vi "I2C FPGA.vi"() -> ()   [LabVIEW 2017]
uses:
  <vilib>/IEDriver/SPIandI2C/FPGA/Library/IP SPI&I2C.lvlib
  <vilib>/IEDriver/SPIandI2C/FPGA/Private/Configure Port (I2C).vi
  <vilib>/IEDriver/SPIandI2C/FPGA/Private/Read Port (I2C).vi
  <vilib>/IEDriver/SPIandI2C/FPGA/Private/Arm Port (I2C).vi
  <vilib>/IEDriver/SPIandI2C/FPGA/Private/Write Port (I2C).vi
  <vilib>/IEDriver/SPIandI2C/FPGA/Private/Initialize Port (I2C).vi
  <vilib>/IEDriver/SPIandI2C/FPGA/Private/IP Port (I2C).vi
  <vilib>/eio/EIONode/EIONode.xnode
  <vilib>/rvi/eio/common/nirviEmuTemplateMethod_errors.vi
panel:
  in  "I2C Protocol Action 0":T1(ring)=enum."Idle"
  in  "I2C Protocol Input Data 0":u8
  out "I2C Protocol Output Data 0":u8
  in  "I2C Protocol Configure 0":T2 {"Command (Write & Read)" items=["Write & Read", "Write", "Read"]}
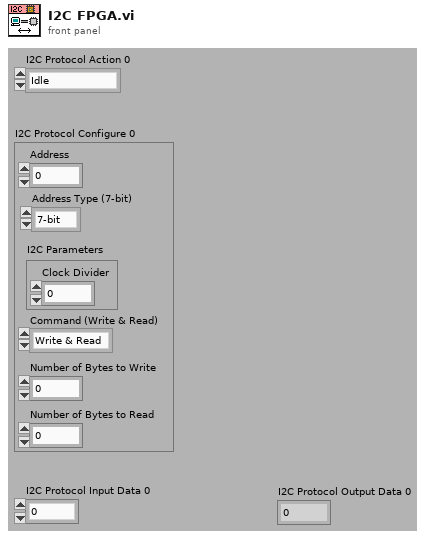
[diagram p1: front panel]
types:
  T1 = enum8{"Configure", "Write", "Arm", "Read", "Set Idle", "Idle"}
  T2 = cluster{"Address":u16, "Address Type (7-bit)":enum16{"7-bit", "10-bit"}, "I2C Parameters":cluster{"Clock Divider":u32}, "Command (Write & Read)":u8, "Number of Bytes to Write":u16, "Number of Bytes to Read":u16}
  T3 = typedef "IP SPI&I2C.lvlib/Private Data (I2C).ctl" = cluster{"Arm Trigger":refnum<k21>, "API to IP Data":refnum<k21>, "IP to API Data":refnum<k21>, "Configuration Register":refnum<k21>, "Configuration Lock":refnum<k21>}
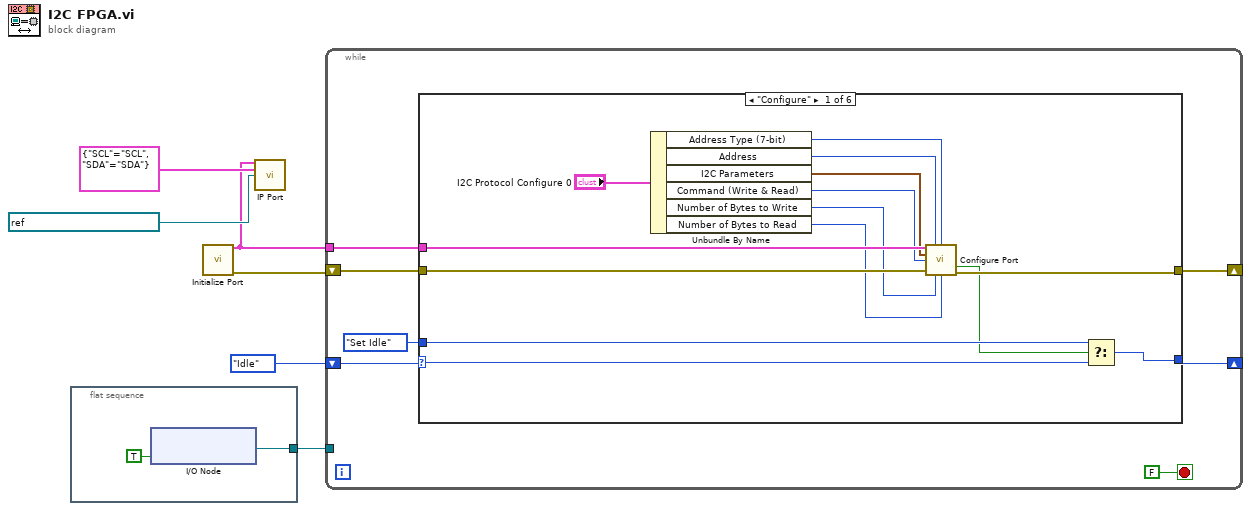
[diagram p0: block diagram]
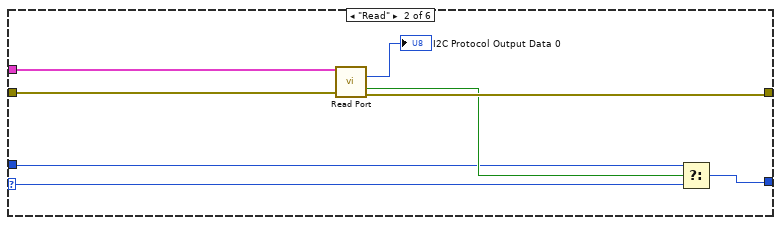
[diagram p2: hidden frame]
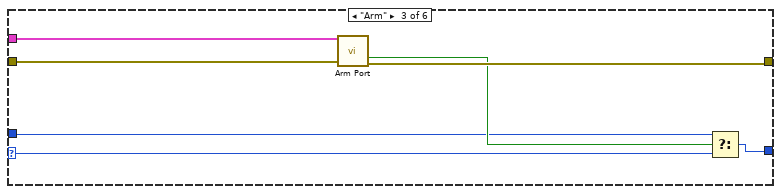
[diagram p3: hidden frame]
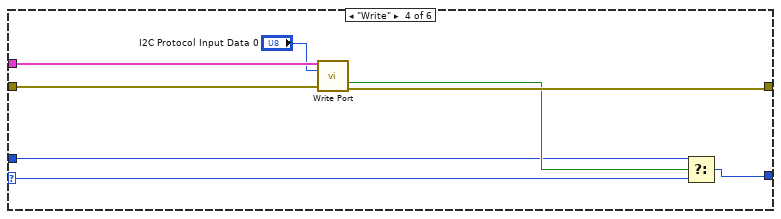
[diagram p4: hidden frame]
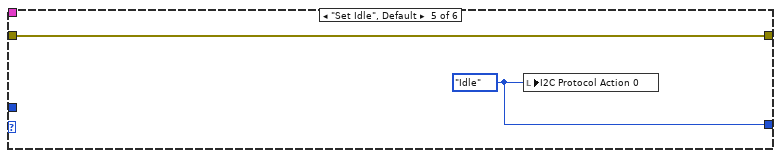
[diagram p5: hidden frame]
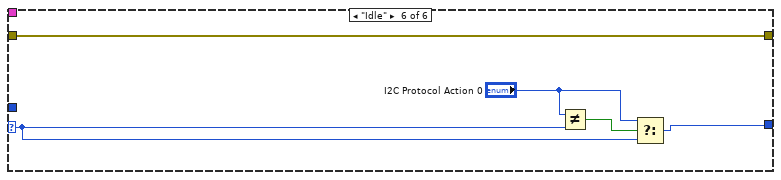
[diagram p6: hidden frame]
diagram:
  n1 = flat-sequence {
    tunnel: [w7] -> w1
    frame #0 {
      n2 = xnode "I/O Node"("Mod1/DIO1"=TRUE) -> ("FPGA I/O Out"=w7:refnum<k21>)  [unwired: 1 in]
    }
  }
  n3 = call-poly <vilib>:"Initialize Port.vi"() -> ("Private Data Out"=w4:T3, "error out"=w3:errorcluster)  [unwired: 14 in]
  n4 = call-poly <vilib>:"IP Port.vi"("Private Data In"=w4, "I2C FPGA IO"=cluster{"SCL":refnum<k21>, "SDA":refnum<k21>} {"SCL"="SCL", "SDA"="SDA"}, "FPGA Clock"=refnum<k21> "40 MHz Onboard Clock") -> ()  [unwired: 13 in]
  n5 = while {
    shift-right: [w12] -> _
    shift-left: w3 -> [w14]
    tunnel: w4 -> [w15]
    shift-right: [w10] -> _
    shift-left: T1."Idle" ("Action") -> [w11]
    tunnel: w1 -> [_]
    stop <- FALSE stop-if-true
    n6 = case shown="\"Configure\"" w11 {
      selector: w11 -> [w20 w31 w39 w46 _ w56]
      tunnel: w15 -> [w29 w37 w44 w52 _ _]
      tunnel: w14 -> [w28 w36 w43 w51 w54 w59]
      tunnel: [w27 w35 w42 w50 w54 w59] -> w12
      tunnel: [w21 w33 w41 w47 w53 w55] -> w10
      tunnel: T1."Set Idle" ("Action") -> [w19 w30 w38 w45 _ _]
      frame "Configure" {
        n7 = Unbundle By Name("I2C Protocol Configure 0") -> ("Address Type (7-bit)"=w25:enum16{"7-bit", "10-bit"}, "Address"=w16:u16, "I2C Parameters"=w24:cluster{"Clock Divider":u32}, "Command (Write & Read)"=w17:u8, "Number of Bytes to Write"=w23:u16, "Number of Bytes to Read"=w22:u16)
        n8 = call-poly <vilib>:"Configure Port.vi"("Private Data In"=w29, "Address"=w16, "Address Type (7-bit)"=w25, "I2C Parameters"=w24, "Command (Write & Read)"=w17, "error in"=w28, "Number of Bytes to Write"=w23, "Number of Bytes to Read"=w22) -> ("Done"=w18:bool, "error out"=w27:errorcluster)  [unwired: 5 in, 1 out]
        n9 = Select(t=w19, s=w18, f=w20) -> (s? t:f=w21:T1)
      }
      frame "Read" {
        n10 = call-poly <vilib>:"Read Port.vi"("Private Data In"=w37, "error in"=w36) -> ("Data Out"=→"I2C Protocol Output Data 0":u8, "Output Valid"=w32:bool, "error out"=w35:errorcluster)  [unwired: 10 in, 1 out]
        n11 = Select(t=w30, s=w32, f=w31) -> (s? t:f=w33:T1)
      }
      frame "Arm" {
        n12 = call-poly <vilib>:"Arm Port.vi"("Private Data In"=w44, "error in"=w43) -> ("Done"=w40:bool, "error out"=w42:errorcluster)  [unwired: 11 in, 1 out]
        n13 = Select(t=w38, s=w40, f=w39) -> (s? t:f=w41:T1)
      }
      frame "Write" {
        n14 = call-poly <vilib>:"Write Port.vi"("Private Data In"=w52, "Data In"="I2C Protocol Input Data 0", "error in"=w51) -> ("Done"=w48:bool, "error out"=w50:errorcluster)  [unwired: 10 in, 1 out]
        n15 = Select(t=w45, s=w48, f=w46) -> (s? t:f=w47:T1)
      }
      frame "Set Idle", Default {
        w53 = T1."Idle" ("Action")
        n16 = local write "I2C Protocol Action 0"(w53) -> ()
      }
      frame "Idle" {
        n17 = Not Equal?(x="I2C Protocol Action 0", y=w56) -> (x != y?=w58:bool)
        n18 = Select(t="I2C Protocol Action 0", s=w58, f=w56) -> (s? t:f=w55:T1)
      }
    }
  }
